vi "HRM-share_error.vi"(8 "error in (no error)":errorcluster, 9 "module name":string, 11 "Init cluster":T1) -> (0 "error out":errorcluster)   [LabVIEW 2020]
uses:
  HRM-Stage4-init_cluster.ctl
  HRM-stage4-config_data.ctl
  HRM-Stage4-User_events.ctl
  process/HRM-process-peak_detect_setting.ctl
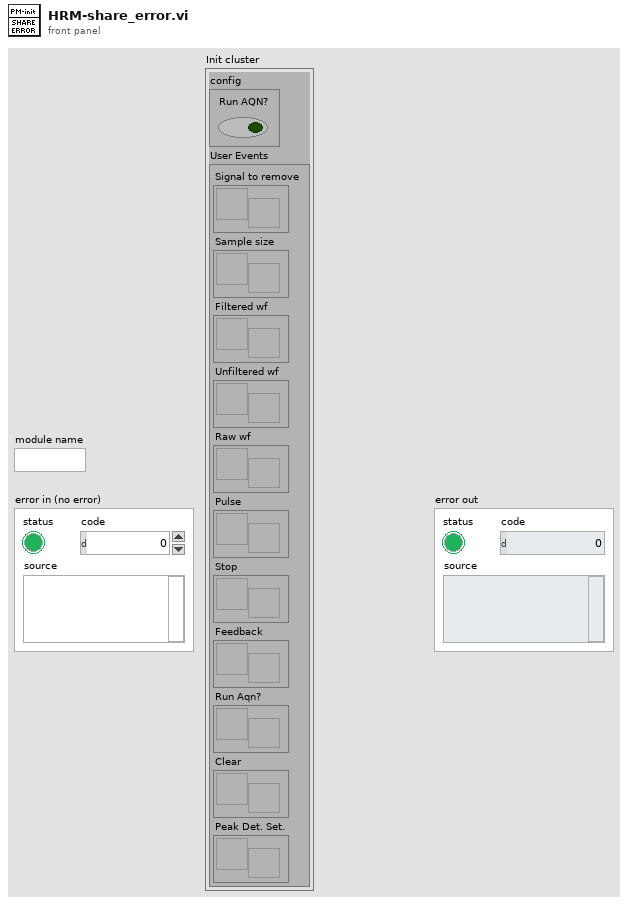
[diagram p1: front panel]
types:
  T1 = typedef "HRM-Stage4-init_cluster.ctl" = cluster{"config":T2, "User Events":T3}
  T2 = typedef "HRM-stage4-config_data.ctl" = cluster{"Run AQN?":bool}
  T3 = typedef "HRM-Stage4-User_events.ctl" = cluster{"Signal to remove":refnum<user-event>, "Sample size":refnum<user-event>, "Filtered wf":refnum<user-event>, "Unfiltered wf":refnum<user-event>, "Raw wf":refnum<user-event>, "Pulse":refnum<user-event>, "Stop":refnum<user-event>, "Feedback":refnum<user-event>, "Run Aqn?":refnum<user-event>, "Clear":refnum<user-event>, "Peak Det. Set.":refnum<user-event>}
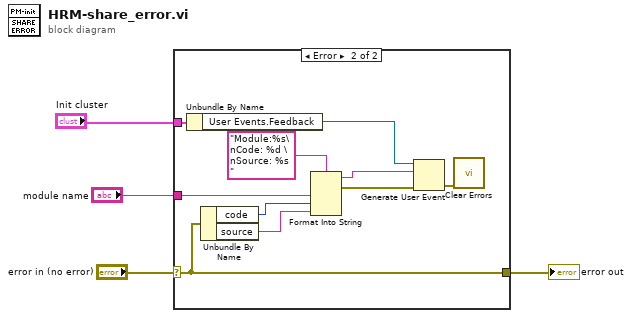
[diagram p0: block diagram]
diagram:
  n1 = case shown="Error" "error in (no error)" {
    selector: "error in (no error)" -> [w5 w6]
    tunnel: "Init cluster" -> [_ w15]
    tunnel: "module name" -> [_ w9]
    tunnel: [w5 w6] -> w2
    frame No Error {
    }
    frame Error {
      n2 = Unbundle By Name(w15) -> ("User Events.Feedback"=w14:refnum<user-event>)
      n3 = Unbundle By Name(w6) -> ("code"=w10:i32, "source"=w11:string)
      n4 = Format Into String(format string="Module:%s\nCode: %d \nSource: %s ", w9, w10, w11) -> (resulting string=w8:string, error out=w7:errorcluster)  [unwired: 2 in]
      n5 = Generate User Event(user event=w14, event data cluster=w8, error in=w7) -> (error out=w13:errorcluster)  [unwired: 1 in, 1 out]
      n6 = call <vilib>:"Clear Errors.vi"("error in (no error)"=w13) -> ()  [unwired: 5 in, 2 out]
    }
  }
  "error out" <- w2
